vi "FoodCheck.vi"(8 "error in (no error)":errorcluster, 9 "IterationNumber":i32, 11 "Snake in":refnum<class "Snake.lvclass">) -> (0 "error out":errorcluster, 3 "Snake out":refnum<class "Snake.lvclass">)   [LabVIEW 2014, in "Snake.lvclass"]
uses:
  Snake.lvclass
  Snake.lvclass/Snake.ctl
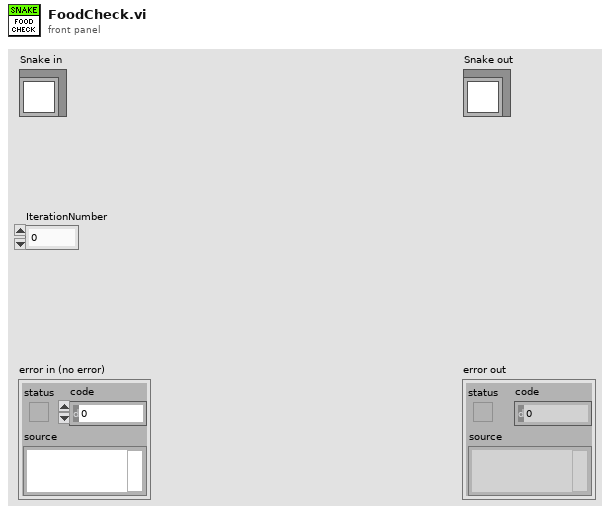
[diagram p1: front panel]
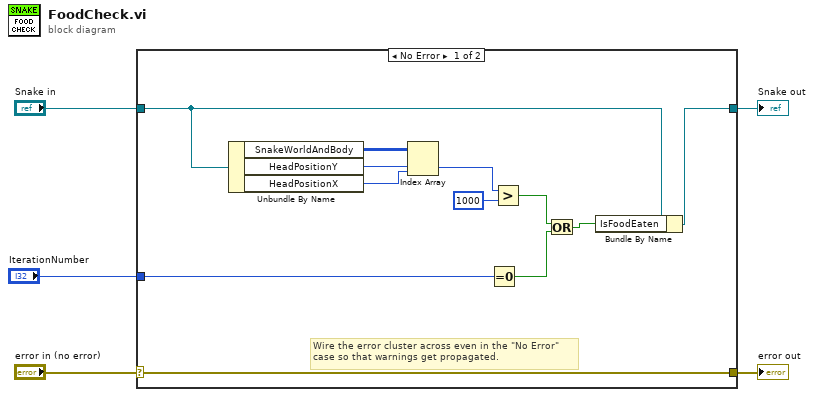
[diagram p0: block diagram]
diagram:
  n1 = case shown="No Error" "error in (no error)" {
    selector: "error in (no error)" -> [w17 w19]
    tunnel: [w17 w19] -> w4
    tunnel: [w8 w18] -> w2
    tunnel: "Snake in" -> [w16 w18]
    tunnel: "IterationNumber" -> [w7 _]
    frame No Error {
      # "Wire the error cluster across even in the \"No Error\"\ncase so that warnings get propagated."
      n2 = Unbundle By Name(w16) -> ("SnakeWorldAndBody"=w15:u32[][], "HeadPositionY"=w14:i32, "HeadPositionX"=w13:i32)
      n3 = Index Array(array=w15, index (row)=w14, index (col)=w13) -> (element=w12:u32)
      n4 = Equal To 0?(x=w7) -> (x = 0?=w9:bool)
      n5 = Greater?(x=w12, y=u32 1000) -> (0:w10:bool)
      n6 = Or(x=w10, y=w9) -> (x .or. y?=w6:bool)
      n7 = Bundle By Name(cluster=w16, "IsFoodEaten"=w6) -> (w8:refnum<class "Snake.lvclass">)
    }
    frame Error {
    }
  }
  "error out" <- w4
  "Snake out" <- w2
